vi "MasterAquisitionFile_NoLiveDisplays_IOS.vi"() -> ()   [LabVIEW 2018]
uses:
  <vilib>/userdefined/High Color/IMAQdx.ctl
  <vilib>/vision/driver/IMAQdx.llb/IMAQdx Camera Control Mode.ctl
  <vilib>/vision/driver/IMAQdx.llb/IMAQdx Acquisition Mode.ctl
  <vilib>/vision/driver/IMAQdx.llb/IMAQdx Buffer Number Mode.ctl
  <vilib>/DAQmx/write.llb/DAQmx Write (Digital Bool 1Line 1Point).vi
  <vilib>/DAQmx/read.llb/DAQmx Read (Analog 1D Wfm NChan NSamp).vi
  <vilib>/DAQmx/write.llb/DAQmx Write (Digital 1D Bool NChan 1Samp 1Line).vi
  <vilib>/DAQmx/create/channels.llb/DAQmx Create Channel (DO-Digital Output).vi
  <vilib>/DAQmx/create/channels.llb/DAQmx Create Channel (CO-Pulse Generation-Frequency).vi
  <vilib>/DAQmx/configure/timing.llb/DAQmx Timing (Implicit).vi
  <vilib>/DAQmx/create/channels.llb/DAQmx Create Channel (AI-Voltage-Basic).vi
  <vilib>/DAQmx/configure/timing.llb/DAQmx Timing (Sample Clock).vi
  <vilib>/DAQmx/configure/trigger.llb/DAQmx Start Trigger (Digital Edge).vi
  <vilib>/DAQmx/miscellaneous.llb/DAQmx Fill In Error Info.vi
  <vilib>/vision/driver/NI_Vision_Acquisition_Software.lvlib
  <resource>/objmgr/imaqdx.rc
panel:
  in  "stop":bool
  out "CBV Cam":bool
  out "Pupil Cam":bool
  out "Whisk Cam":bool
  out "Web Cam":bool
  out "Analog Data":bool
  in  "Physical channels":tag="Dev1/ai0:7"
  out "Web Cam Fs":dbl(knob) scale=0.0..200.0
  out "CBV Cam":dbl(knob) scale=0.0..200.0
  out "Whisk Cam Fs":dbl(knob) scale=0.0..200.0
  out "Last Whisk\nBuffer 2":u32=4963
  out "Pupil Cam Fs":dbl(knob) scale=0.0..200.0
  out "Dropped 2":u32(slide) caption="Pupil Cam" scale=0.0..90.0
  in  "Pupil Cam ID":T1="cam2"
  in  "Pupil Cam Trig Source":tag="Dev2/ctr0"
  in  "Exposure Time (microsec)":string="10000"
  out "Solenoids":bool[](array[boolean])
  out "Analog Samples":i32
  in  "Analog Channels":string[](array[string])=["Cortical_LH", "Force_Sensor", "LPadSol", "RPadSol", "AudSol", "Hippocampus", "EMG", "Cortical_RH"]
  in  "Whisker Cam ID":T1="cam1"
  in  "WebCam ID":T1="cam0"
  in  "Analog Acquisition":cluster{"Analog Fs":u16}={"Analog Fs"=20000} {"Analog Fs" format="%0.0f"}
  in  "Camera Acquisition Setup":T2={"CBV Cam Fs"=30, "Whisk Cam Fs"=150, "Web Cam Fs"=15, "Pupil Cam Fs"=30}
  out "Notes Size":i32=7
  out "Notes Reversed":string[](array[string])=["Experimenter", "Animal ID", "Hemisphere", "Solenoid PSI", "Isoflurane time", "Session ID", "Amplifier Gain"]
  out "Notes Array":string[](array[string])=["Amplifier Gain", "Session ID", "Isoflurane time", "Solenoid PSI", "Hemisphere", "Animal ID", "Experimenter"]
  in  "Notes:":T3={"Experimenter"="Kevin", "Animal ID"="T103", "Hemisphere"="Both", "Solenoid PSI"="10", "Isoflurane time"="1000", "Session ID"="Imaging Session One", "Amplifier Gain"="10000"}
  in  "Whisk Cam Trig Source":tag="Dev1/ctr1"
  in  "CBV Cam Trig Source":tag="Dev1/ctr0"
  in  "Left Pad":tag="Dev1/port0/line0"
  in  "Right Pad":tag="Dev1/port0/line1"
  in  "Auditory":tag="Dev1/port0/line2"
  in  "Offset (s)":dbl=15.0
  in  "Duration (s)":dbl=0.1 step=0.1
  in  "Interval (s)":dbl=30.0
  in  "Right Pad":dbl=1.0
  in  "Left Pad":dbl=1.0
  in  "Auditory":dbl=1.0
  in  "Target Path":path=path "D:/T103/Imaging Session One 8.2.19" caption="Final saved file location"
  out "Dropped":u32(slide) caption="Whisk Cam" scale=0.0..450.0
  out "Current file name":string="190412_14_35_08"
  out "CBV Camera":bool
  out "Time Elapsed (Min)":cluster{dbl, dbl}(slide)={15.0, 0.0} scale=0.0..15.0 scale format="%#_2g"
  in  "Time (min)":dbl(knob)=15.0 min=0.5 max=20.0 step=0.5 scale=0.0..20.0 scale format="%#_2g"
  in  "Temp Path":path=path "D:/LabVIEW Streamed Data" caption="Temporary path for streamed data"
  out "Last CBV\nBuffer":i32=9926
  out "Last Whisk\nBuffer":u32=49638
  # "Stimuli"
  # "LPAD"
  # "RPAD"
  # "AUD"
  # "Whisk Cam ID"
  # "Pupil Cam ID"
  # "Ratio"
  # "Web Cam ID"
  # "Data Sampling Rates"
  # "Ratio"
  # "Ratio"
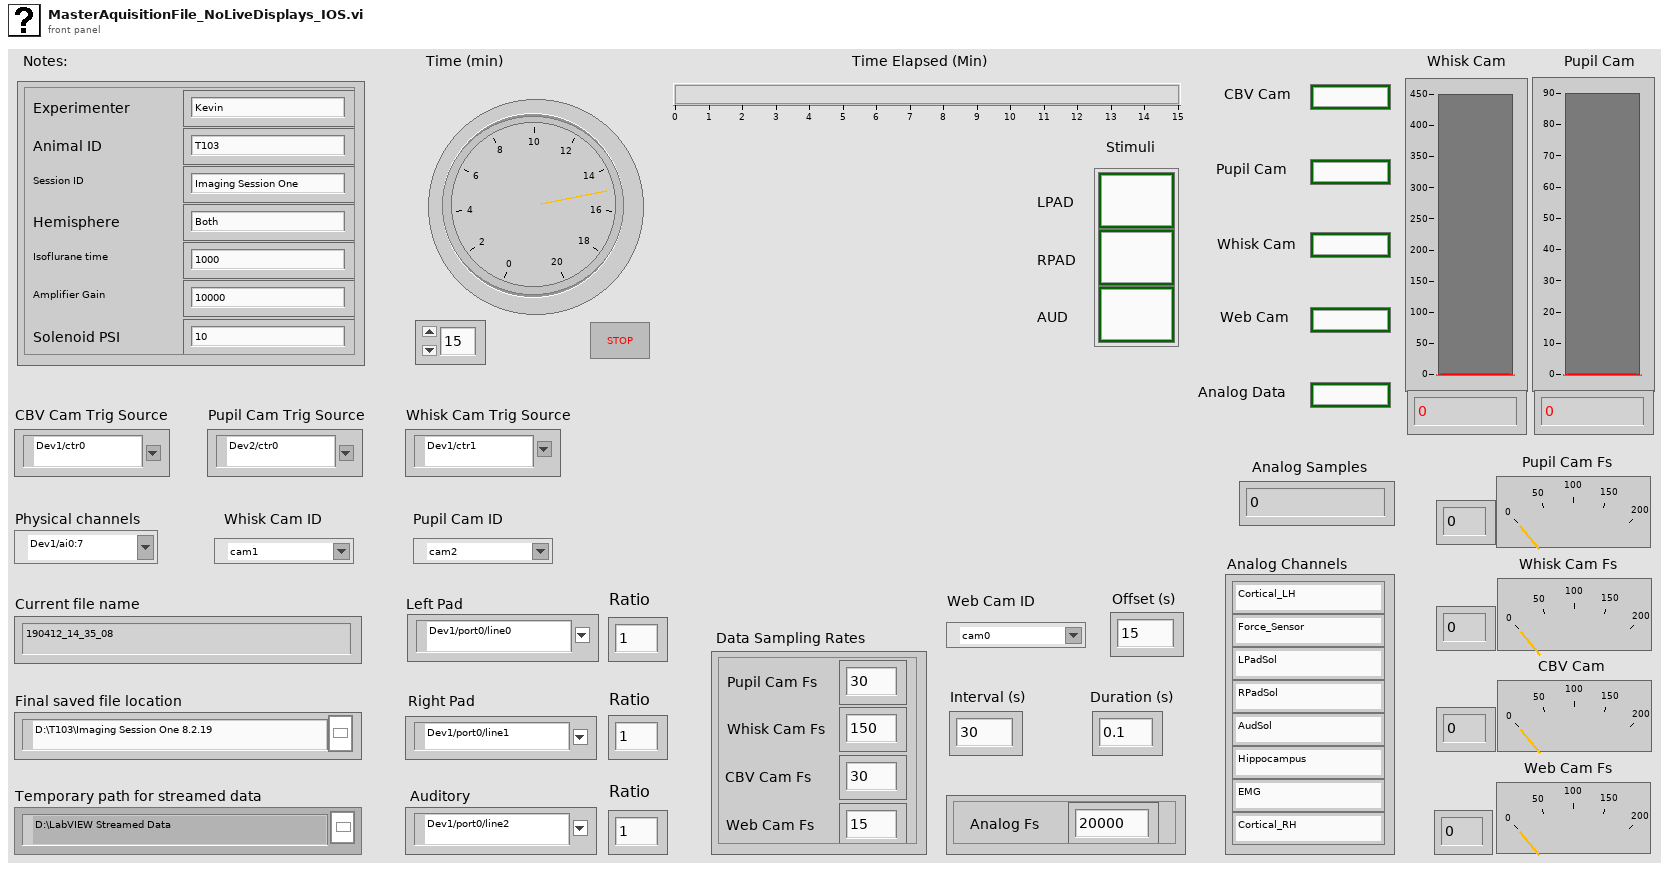
[diagram p1: front panel]
types:
  T1 = typedef "IMAQdx.ctl" = refnum<k21>
  T2 = cluster{"CBV Cam Fs":u16, "Whisk Cam Fs":u16, "Web Cam Fs":u16, "Pupil Cam Fs":u16}
  T3 = cluster{"Experimenter":string, "Animal ID":string, "Hemisphere":string, "Solenoid PSI":string, "Isoflurane time":string, "Session ID":string, "Amplifier Gain":string}
  T4 = enum16{"open", "replace", "create", "open or create", "replace or create", "replace or create with confirmation"}
  T5 = typedef "Image Type" = u32
  T6 = typedef "NI_Vision_Acquisition_Software.lvlib/IMAQdx Acquisition Mode.ctl" = enum32{"One Shot", "Continuous"}
  T7 = typedef "NI_Vision_Acquisition_Software.lvlib/IMAQdx Camera Control Mode.ctl" = enum32{"Controller", "Listener"}
  T8 = enum16{"open", "open or create", "create or replace", "create", "open (read-only)"}
  T9 = typedef "IMAQ AVI2 Refnum.ctl" = refnum<k20>
  T10 = typedef "IMAQ Image.ctl" = refnum<image>
  T11 = enum16{"big-endian, network order", "native, host order", "little-endian"}
  T12 = typedef "NI_Vision_Acquisition_Software.lvlib/IMAQdx Buffer Number Mode.ctl" = enum32{"Next", "Last", "Buffer Number", "Every", "Last New"}
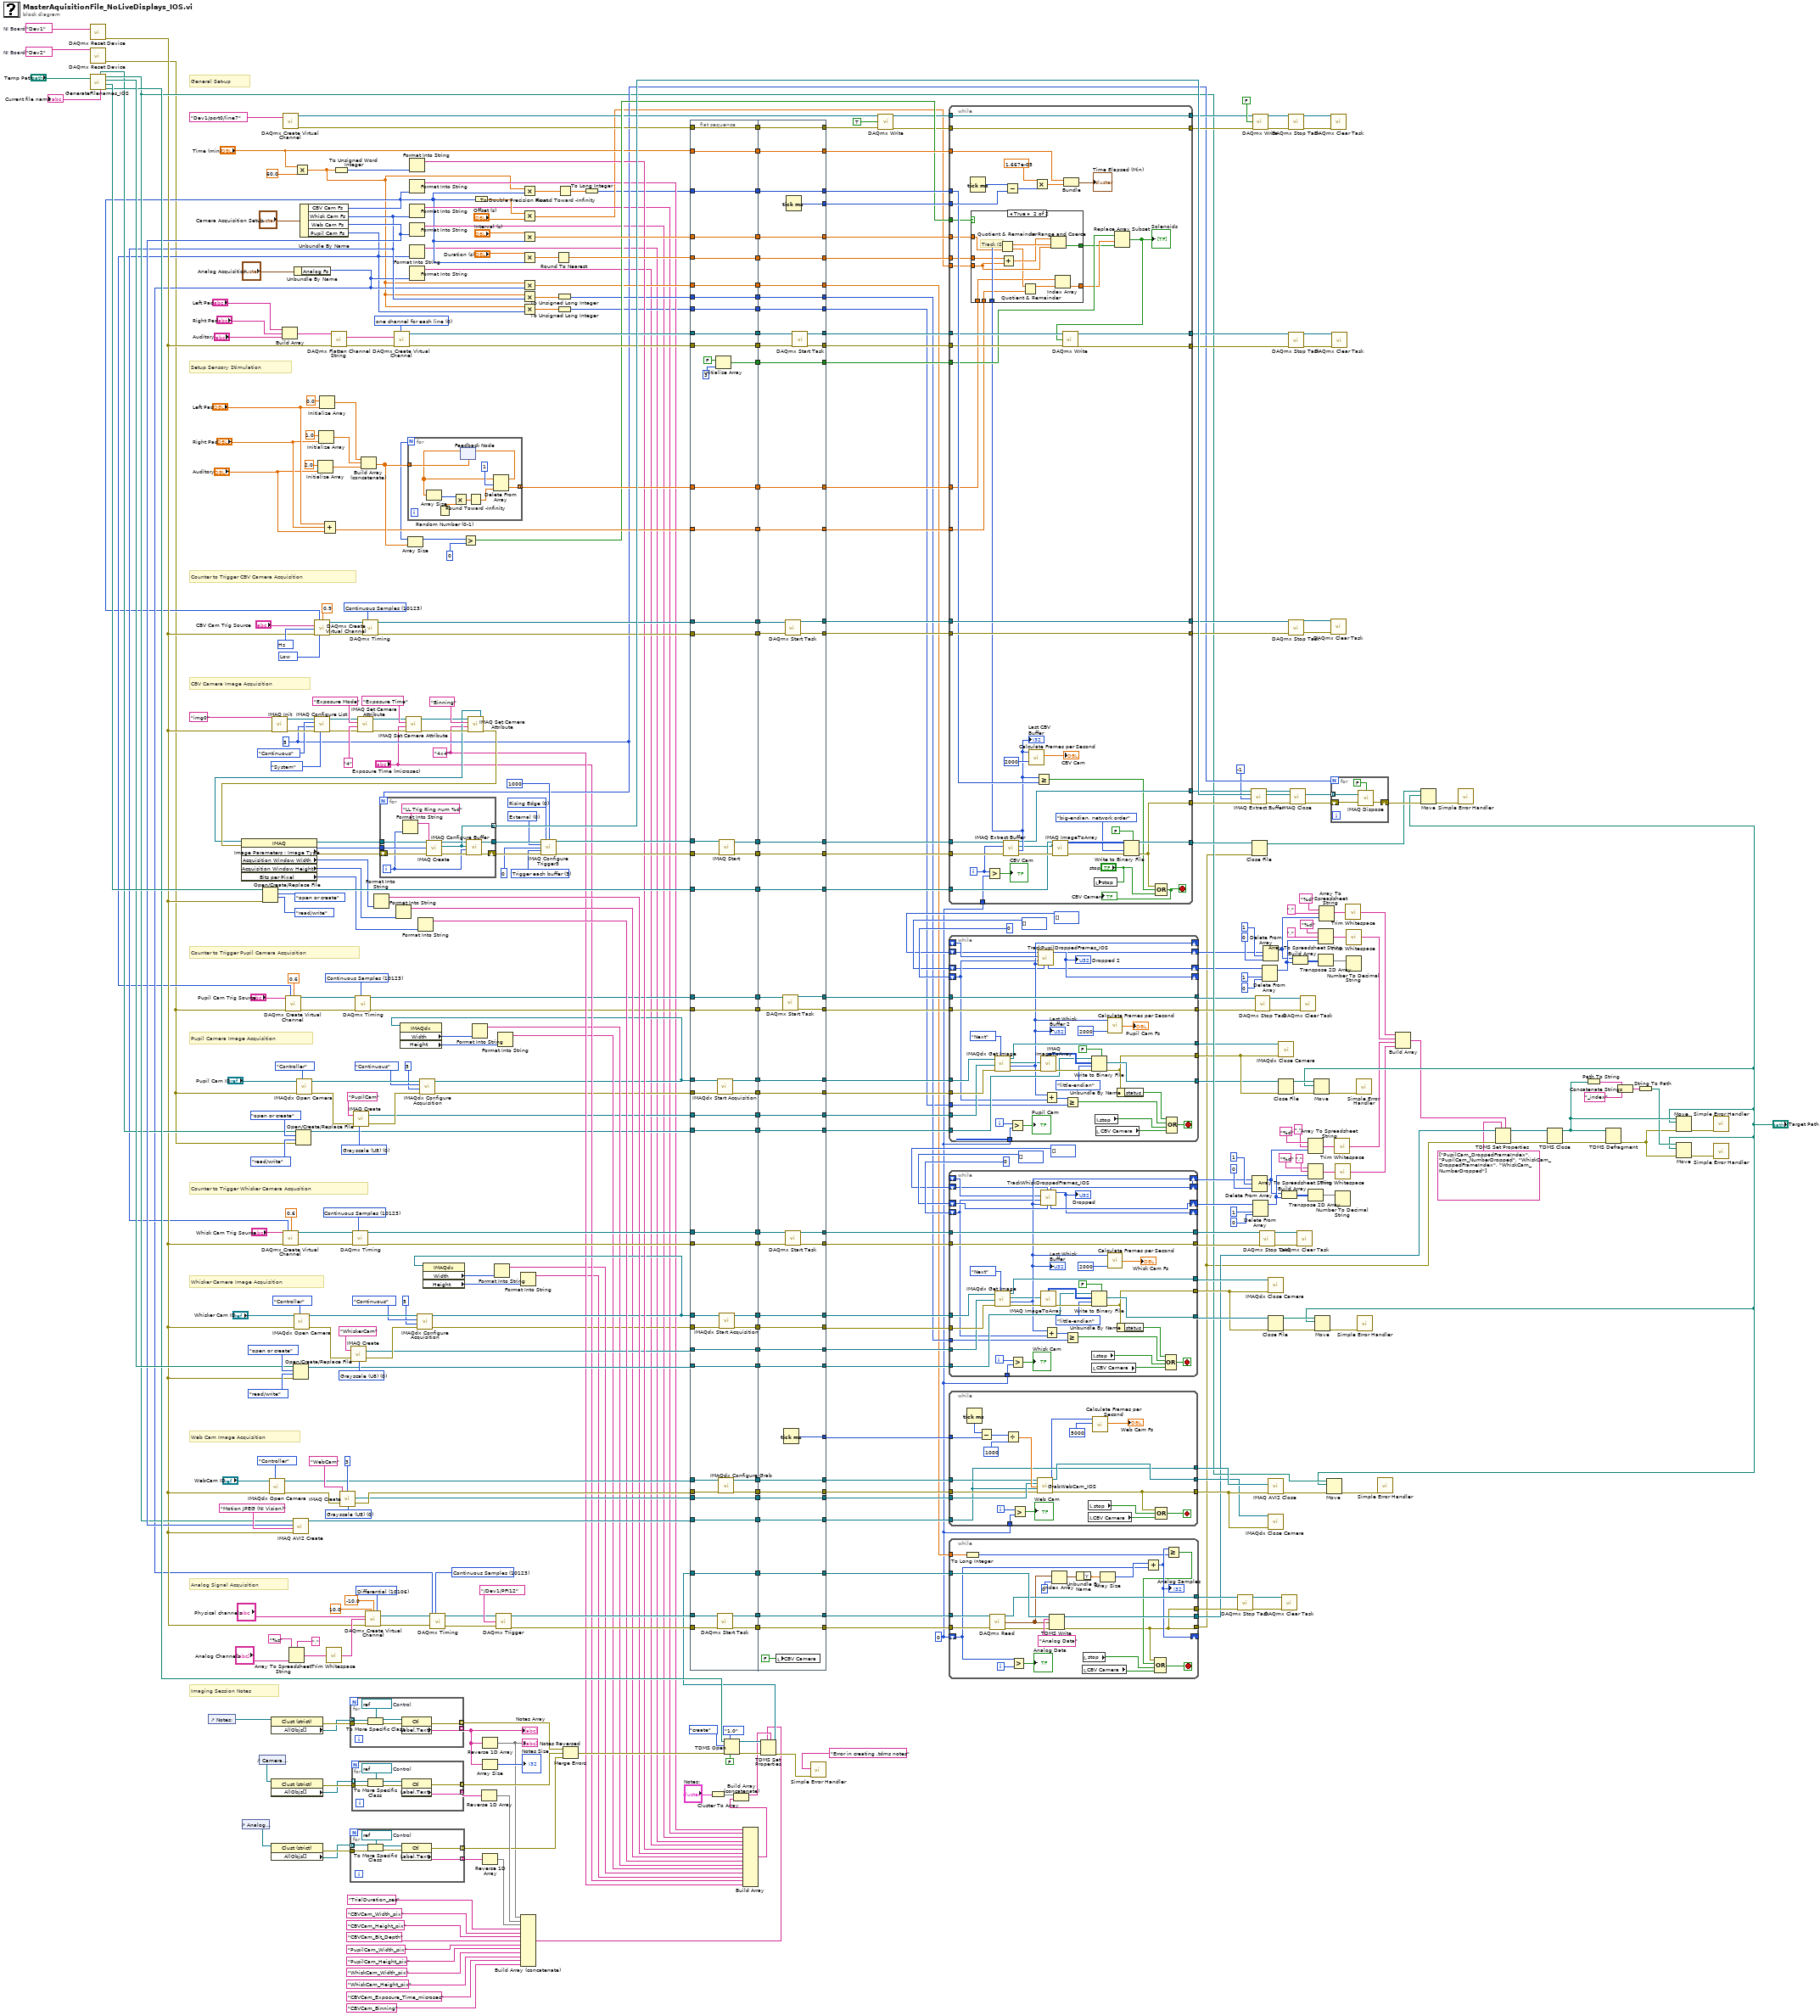
[diagram p0: block diagram]
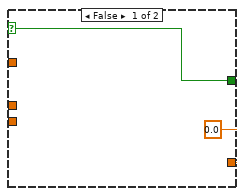
[diagram p2: hidden frame]
diagram:
  w17 = tag "Dev2"  # NI Board
  w108 = 10123 items=["Finite Samples"=10178, "Continuous Samples"=10123, "Hardware Timed Single Point"=12522] ("sample mode")
  w115 = T5 0 items=["Grayscale (U8)", "Grayscale (I16)", "Grayscale (SGL)", "Complex (CSG)", "RGB (U32)", "HSL (U32)", "RGB (U64)", "Grayscale (U16)"] ("Image Type")
  w97 = "4x4" ("Attribute Value")
  w23 = 0
  w281 = 0 items=["one channel for each line", "one channel for all lines"] ("line grouping")
  w334 = 10123 items=["Finite Samples"=10178, "Continuous Samples"=10123, "Hardware Timed Single Point"=12522] ("sample mode")
  w337 = 10106 items=["default"=-1, "RSE"=10083, "NRSE"=10078, "Differential"=10106, "Pseudodifferential"=12529] ("input terminal configuration")
  w388 = T5 0 items=["Grayscale (U8)", "Grayscale (I16)", "Grayscale (SGL)", "Complex (CSG)", "RGB (U32)", "HSL (U32)", "RGB (U64)", "Grayscale (U16)"] ("Image Type")
  w408 = u32 0 items=["Rising Edge", "Falling Edge"] ("Trigger Polarity")
  w411 = u32 0 items=["External"=0, "RTSI"=1, "ISO In"=2, "Scaled Encoder"=5] ("Trigger Type")
  w402 = tag "Dev1"  # NI Board
  w403 = 10123 items=["Finite Samples"=10178, "Continuous Samples"=10123, "Hardware Timed Single Point"=12522] ("sample mode")
  w406 = 10373 items=["Hz"=10373] ("units")
  w407 = 10214 items=["High"=10192, "Low"=10214] ("idle state")
  w127 = u32 5 ("Number of Buffers")
  w409 = u32 3 items=["Disabled", "Trigger start of acquisition", "Trigger start of each buffer list", "Trigger each buffer", "Trigger each line (linescan)", "Trigger end of acquisition"] ("Action")
  w423 = 10123 items=["Finite Samples"=10178, "Continuous Samples"=10123, "Hardware Timed Single Point"=12522] ("sample mode")
  w430 = T5 0 items=["Grayscale (U8)", "Grayscale (I16)", "Grayscale (SGL)", "Complex (CSG)", "RGB (U32)", "HSL (U32)", "RGB (U64)", "Grayscale (U16)"] ("Image Type")
  # "General Set-up"
  # "Pupil Camera Image Acquisition"
  # "Counter to Trigger Pupil Camera Acquisition"
  # "Whisker Camera Image Acquisition"
  # "Imaging Session Notes"
  # "Setup Sensory Stimulation"
  # "CBV Camera Image Acquisition"
  # "Counter to Trigger CBV Camera Acquisition"
  # "Counter to Trigger Whisker Camera Acqusition"
  # "Web Cam Image Acquisition"
  # "Analog Signal Acquisition"
  n1 = call <vilib>:"DAQmx Reset Device.vi"("device in"=w402) -> ("error out"=w82:errorcluster)  [unwired: 14 in]
  n2 = call <vilib>:"DAQmx Reset Device.vi"("device in"=w17) -> ("error out"=w16:errorcluster)  [unwired: 14 in]
  n3 = call "GenerateFilenames_IOS.vi"("path"="Temp Path") -> ("TDMS Path"=w237:path, "Dalsa Path"=w395:path, "Basler Path"=w391:path, "WebCam Path"=w126:path, "Analog file name"=→"Current file name":string, "Basler2 Path"=w106:path)  [unwired: 5 in]
  n4 = control-ref of="Notes:"() -> (w242:refnum<vi>)
  n5 = control-ref of="Analog Acquisition"() -> (w220:refnum<vi>)
  n6 = control-ref of="Camera Acquisition Setup"() -> (w221:refnum<vi>)
  n7 = Open/Create/Replace File(file path (use dialog)=w395, error in=w82, operation (0:open)=T4."open or create", access (0:read/write)=enum16{"read/write", "read-only", "write-only"}."read/write") -> (refnum out=w338:refnum<file>)  [unwired: 2 in, 2 out]
  n8 = call <vilib>:"IMAQdx Open Camera.vi"("Camera Control Mode"=IMAQdx_Camera_Control_Mode."Controller", "error in"=w82, "Session In"="WebCam ID") -> ("error out"=w384:errorcluster, "Session Out"=w382:T1)  [unwired: 7 in]
  n9 = property class="Clust (strict)"(reference=w242) -> (error out=w245:errorcluster, "AllObjs[]"=w134:refnum<vi>[])  [unwired: 1 in, 1 out]
  n10 = property class="Clust (strict)"(reference=w221) -> (error out=w240:errorcluster, "AllObjs[]"=w135:refnum<vi>[])  [unwired: 1 in, 1 out]
  n11 = property class="Clust (strict)"(reference=w220) -> (error out=w219:errorcluster, "AllObjs[]"=w133:refnum<vi>[])  [unwired: 1 in, 1 out]
  n12 = call <vilib>:"IMAQ Init.vi"("error in (no error)"=w82, "Interface Name"="img0") -> ("error out"=w421:errorcluster, "IMAQ Session Out"=w422:refnum<k11>)  [unwired: 8 out]
  n13 = Build Array("Left Pad", "Right Pad", "Auditory") -> (w9:tag[])
  n14 = call-poly <vilib>:"DAQmx Create Virtual Channel.vi"("lines"=tag "Dev1/port0/line7") -> ("task out"=w167:refnum<k21>, "error out"=w170:errorcluster)  [unwired: 13 in]
  n15 = Array To Spreadsheet String(delimiter (Tab)=",", array="Analog Channels", 3:"%s" ("format string")) -> (spreadsheet string=w206:string)
  n16 = Open/Create/Replace File(file path (use dialog)=w391, error in=w82, operation (0:open)=T4."open or create", access (0:read/write)=enum16{"read/write", "read-only", "write-only"}."read/write") -> (refnum out=w356:refnum<file>)  [unwired: 2 in, 2 out]
  n17 = Unbundle By Name("Analog Acquisition") -> ("Analog Fs"=w63:u16)
  n18 = call <vilib>:"IMAQdx Open Camera.vi"("Camera Control Mode"=IMAQdx_Camera_Control_Mode."Controller", "error in"=w82, "Session In"="Whisker Cam ID") -> ("error out"=w433:errorcluster, "Session Out"=w436:T1)  [unwired: 7 in]
  n19 = Multiply(x="Time (min)", y=60.0) -> (x*y=w25:dbl)
  n20 = Open/Create/Replace File(file path (use dialog)=w106, error in=w16, operation (0:open)=T4."open or create", access (0:read/write)=enum16{"read/write", "read-only", "write-only"}."read/write") -> (refnum out=w87:refnum<file>)  [unwired: 2 in, 2 out]
  n21 = call <vilib>:"IMAQdx Open Camera.vi"("Camera Control Mode"=IMAQdx_Camera_Control_Mode."Controller", "error in"=w16, "Session In"="Pupil Cam ID") -> ("error out"=w118:errorcluster, "Session Out"=w121:T1)  [unwired: 7 in]
  n22 = Unbundle By Name("Camera Acquisition Setup") -> ("CBV Cam Fs"=w27:u16, "Whisk Cam Fs"=w68:u16, "Web Cam Fs"=w214:u16, "Pupil Cam Fs"=w61:u16)
  n23 = call-poly <vilib>:"DAQmx Create Virtual Channel.vi"("frequency"=w68, "duty cycle"=0.6, "counter"="Whisk Cam Trig Source", "error in"=w82) -> ("task out"=w425:refnum<k21>, "error out"=w424:errorcluster)  [unwired: 10 in]
  n24 = call-poly <vilib>:"DAQmx Create Virtual Channel.vi"("frequency"=w61, "duty cycle"=0.6, "counter"="Pupil Cam Trig Source", "error in"=w16) -> ("task out"=w110:refnum<k21>, "error out"=w109:errorcluster)  [unwired: 10 in]
  n25 = call "IMAQ AVI2 Create"("error in (no error)"=w82, "Codec"="Motion JPEG (NI Vision)", "Frames Per Second"=w214, "AVI Path"=w126) -> ("AVI Refnum"=w374:T9)  [unwired: 6 in, 1 out]
  n26 = call <vilib>:"IMAQ Configure List.vi"("Memory Location"=enum16{"System", "Onboard"}."System", "error in (no error)"=w421, "Number of buffers"=w127, "Continuous?"=enum16{"One-Shot", "Continuous"}."Continuous" ("Continuous ?"), "IMAQ Session In"=w422) -> ("error out"=w148:errorcluster, "IMAQ Session Out"=w144:refnum<k11>)  [unwired: 1 in, 4 out]
  n27 = call-poly <vilib>:"DAQmx Create Virtual Channel.vi"("frequency"=w27, "duty cycle"=0.9, "counter"="CBV Cam Trig Source", "units"=w406, "error in"=w82, "idle state"=w407) -> ("task out"=w405:refnum<k21>, "error out"=w404:errorcluster)  [unwired: 8 in]
  n28 = Initialize Array(2.0 ("element"), "Auditory") -> (w21:dbl[])
  n29 = Initialize Array(1.0 ("element"), "Right Pad") -> (w285:dbl[])
  n30 = Initialize Array(0.0 ("element"), "Left Pad") -> (w286:dbl[])
  n31 = Compound Arithmetic op=ADD("Left Pad", "Right Pad", "Auditory") -> (w265:dbl)
  n32 = call <vilib>:"Trim Whitespace.vi"("string"=w206) -> ("trimmed string"=w205:string)  [unwired: 1 in]
  n33 = call <vilib>:"DAQmx Flatten Channel String.vi"("names in"=w9, "error in"=w82) -> ("names out"=w247:string, "error out"=w246:errorcluster)  [unwired: 12 in]
  n34 = To Unsigned Word Integer(number=w25) -> (unsigned 16bit integer=w200:u16)
  n35 = call "IMAQ Create"("Border Size"=3, "Image Name"="WebCam", "Image Type"=w388, "error in (no error)"=w384) -> ("New Image"=w381:T10, "error out"=w383:errorcluster)  [unwired: 1 in]
  n36 = for {
    tunnel: [w442] -> w244 mode=indexing
    tunnel: w245 -> [w441]
    tunnel: [w439] -> w228 mode=indexing
    tunnel: w134 -> [w438] mode=indexing
    w443 = refnum<vi> refnum  # Control
    n37 = To More Specific Class(target class=w443, reference=w438, error in=w441) -> (specific class reference=w444:refnum<vi>, error out=w440:errorcluster)
    n38 = property class="Ctl"(reference=w444, error in=w440) -> (error out=w439:errorcluster, "Label.Text"=w442:string)  [unwired: 1 out]
  }
  "Notes Array" <- w244
  n39 = for {
    tunnel: [w449] -> w217 mode=indexing
    tunnel: w219 -> [w448]
    tunnel: [w446] -> w218 mode=indexing
    tunnel: w133 -> [w445] mode=indexing
    w450 = refnum<vi> refnum  # Control
    n40 = To More Specific Class(target class=w450, reference=w445, error in=w448) -> (specific class reference=w451:refnum<vi>, error out=w447:errorcluster)
    n41 = property class="Ctl"(reference=w451, error in=w447) -> (error out=w446:errorcluster, "Label.Text"=w449:string)  [unwired: 1 out]
  }
  n42 = call "IMAQ Create"("Image Name"="WhiskerCam", "Image Type"=w430, "error in (no error)"=w433) -> ("New Image"=w187:T10, "error out"=w431:errorcluster)  [unwired: 2 in]
  n43 = for {
    tunnel: [w456] -> w241 mode=indexing
    tunnel: w240 -> [w455]
    tunnel: [w453] -> w227 mode=indexing
    tunnel: w135 -> [w452] mode=indexing
    w457 = refnum<vi> refnum  # Control
    n44 = To More Specific Class(target class=w457, reference=w452, error in=w455) -> (specific class reference=w458:refnum<vi>, error out=w454:errorcluster)
    n45 = property class="Ctl"(reference=w458, error in=w454) -> (error out=w453:errorcluster, "Label.Text"=w456:string)  [unwired: 1 out]
  }
  n46 = call-poly <vilib>:"DAQmx Timing.vi"("task/channels in"=w425, "sample mode"=w423, "error in"=w424) -> ("task out"=w317:refnum<k21>, "error out"=w315:errorcluster)  [unwired: 11 in]
  n47 = call "IMAQ Create"("Image Name"="PupilCam", "Image Type"=w115, "error in (no error)"=w118) -> ("New Image"=w71:T10, "error out"=w116:errorcluster)  [unwired: 2 in]
  n48 = call-poly <vilib>:"DAQmx Timing.vi"("task/channels in"=w110, "sample mode"=w108, "error in"=w109) -> ("task out"=w85:refnum<k21>, "error out"=w83:errorcluster)  [unwired: 11 in]
  n49 = call <vilib>:"IMAQ Set Camera Attribute.vi"("error in (no error)"=w148, "Attribute Value"="4", "Camera Attribute"="Exposure Mode", "IMAQ Session In"=w144) -> ("error out"=w147:errorcluster, "IMAQ Session Out"=w143:refnum<k11>)  [unwired: 4 in]
  n50 = Build Array (concatenate)(w286, w285, w21) -> (w284:dbl[])
  n51 = call-poly <vilib>:"DAQmx Timing.vi"("task/channels in"=w405, "sample mode"=w403, "error in"=w404) -> ("task out"=w321:refnum<k21>, "error out"=w319:errorcluster)  [unwired: 11 in]
  n52 = call-poly <vilib>:"DAQmx Create Virtual Channel.vi"("maximum value"=10.0, "minimum value"=-10.0, "input terminal configuration"=w337, "physical channels"="Physical channels", "name to assign"=w205, "error in"=w82) -> ("task out"=w336:refnum<k21>, "error out"=w335:errorcluster)  [unwired: 8 in]
  n53 = call-poly <vilib>:"DAQmx Create Virtual Channel.vi"("lines"=w247, "line grouping"=w281, "error in"=w246) -> ("task out"=w279:refnum<k21>, "error out"=w277:errorcluster)  [unwired: 11 in]
  n54 = call <vilib>:"IMAQ Set Camera Attribute.vi"("error in (no error)"=w147, "Attribute Value"="Exposure Time (microsec)", "Camera Attribute"="Exposure Time", "IMAQ Session In"=w143) -> ("error out"=w146:errorcluster, "IMAQ Session Out"=w142:refnum<k11>)  [unwired: 4 in]
  n55 = Array Size(array=w284) -> (size(s)=w211:i32)
  n56 = for {
    N: w211 -> [_]
    tunnel: w284 -> [w462]
    tunnel: [w459] -> w262 mode=concatenating
    n57 = Random Number (0-1)() -> (number: 0 to 1=w466:dbl)
    n58 = feedback #1(w462) -> (w461:dbl[])
    n59 = Array Size(array=w461) -> (size(s)=w467:i32)
    n60 = Multiply(x=w467, y=w466) -> (x*y=w465:dbl)
    n61 = Round Toward -Infinity(1:w465) -> (0:w464:dbl)
    n62 = Delete From Array(array=w461, length=1, index=w464) -> (deleted portion=w459:dbl[], array with subset deleted=w460:dbl[])
    n63 = feedback-in #1(w460) -> ()
  }
  n64 = Format Into String(w200) -> (resulting string=w202:string)  [unwired: 3 in, 1 out]
  n65 = Format Into String(w27) -> (resulting string=w66:string)  [unwired: 3 in, 1 out]
  n66 = Format Into String(w68) -> (resulting string=w65:string)  [unwired: 3 in, 1 out]
  n67 = Format Into String(w214) -> (resulting string=w64:string)  [unwired: 3 in, 1 out]
  n68 = Format Into String(w61) -> (resulting string=w2:string)  [unwired: 3 in, 1 out]
  n69 = Format Into String(w63) -> (resulting string=w1:string)  [unwired: 3 in, 1 out]
  n70 = call <vilib>:"IMAQdx Configure Acquisition.vi"("error in"=w431, "Number of Buffers"=u32 5, "Continuous?"=IMAQdx_Acquisition_Mode."Continuous", "Session In"=w436) -> ("error out"=w24:errorcluster, "Session Out"=w188:T1)  [unwired: 6 in]
  n71 = call <vilib>:"IMAQdx Configure Acquisition.vi"("error in"=w116, "Number of Buffers"=u32 5, "Continuous?"=IMAQdx_Acquisition_Mode."Continuous", "Session In"=w121) -> ("error out"=w89:errorcluster, "Session Out"=w72:T1)  [unwired: 6 in]
  n72 = property class="IMAQdx"(reference=w72) -> ("Width"=w105:u32, "Height"=w104:u32)  [unwired: 1 in, 2 out]
  n73 = property class="IMAQdx"(reference=w188) -> ("Width"=w199:u32, "Height"=w198:u32)  [unwired: 1 in, 2 out]
  n74 = call-poly <vilib>:"DAQmx Timing.vi"("task/channels in"=w336, "sample mode"=w334, "rate"=w63, "error in"=w335) -> ("task out"=w131:refnum<k21>, "error out"=w333:errorcluster)  [unwired: 10 in]
  n75 = Greater?(x=w211, y=0) -> (0:w209:bool)
  n76 = call <vilib>:"IMAQ Set Camera Attribute.vi"("error in (no error)"=w146, "Attribute Value"=w97, "Camera Attribute"="Binning", "IMAQ Session In"=w142) -> ("error out"=w145:errorcluster, "IMAQ Session Out"=w141:refnum<k11>)  [unwired: 4 in]
  n77 = property class="IMAQ"(reference=w141, error in=w145) -> (reference out=w155:refnum<k11>, error out=w154:errorcluster, "Image Parameters : Image Type"=w417:u32, "Acquisition Window Width"=w197:u32, "Acquisition Window Height"=w196:u32, "Bits per Pixel"=w195:u32)
  n78 = Format Into String(w197) -> (resulting string=w194:string)  [unwired: 3 in, 1 out]
  n79 = for {
    N: w127 -> [_]
    tunnel: [w477] -> w413
    tunnel: w417 -> [w475]
    shift-right: [w476] -> w412
    shift-left: w154 -> [w474]
    tunnel: [w469] -> w414 mode=indexing
    tunnel: w155 -> [w468]
    i -> [w470]
    n80 = Format Into String(format string="LL Trig Ring num %d", w470) -> (resulting string=w472:string)  [unwired: 2 in, 1 out]
    n81 = call "IMAQ Create"("Image Name"=w472, "Image Type"=w475, "error in (no error)"=w474) -> ("New Image"=w469:T10, "error out"=w473:errorcluster)  [unwired: 1 in, 1 out]
    n82 = call <vilib>:"IMAQ Configure Buffer.vi"("error in (no error)"=w473, "Buffer Number"=w470, "Image In"=w469, "IMAQ Session In"=w468) -> ("error out"=w476:errorcluster, "IMAQ Session Out"=w477:refnum<k11>)  [unwired: 2 in, 4 out]
  }
  n83 = Format Into String(w196) -> (resulting string=w128:string)  [unwired: 3 in, 1 out]
  n84 = Format Into String(w195) -> (resulting string=w193:string)  [unwired: 3 in, 1 out]
  n85 = Format Into String(w105) -> (resulting string=w92:string)  [unwired: 3 in, 1 out]
  n86 = To Double Precision Float(number=w27) -> (double precision float=w248:dbl)
  n87 = Reverse 1D Array(array=w241) -> (reversed array=w231:string[])
  n88 = Reverse 1D Array(array=w244) -> (reversed array=w132:string[])
  "Notes Reversed" <- w132
  n89 = Array Size(array=w244) -> (size(s)=→"Notes Size":i32)
  n90 = Reverse 1D Array(array=w217) -> (reversed array=w216:string[])
  n91 = Format Into String(w199) -> (resulting string=w94:string)  [unwired: 3 in, 1 out]
  n92 = call-poly <vilib>:"DAQmx Trigger.vi"("task/channels in"=w131, "source"=tag "/Dev1/PFI12", "error in"=w333) -> ("task out"=w331:refnum<k21>, "error out"=w330:errorcluster)  [unwired: 11 in]
  n93 = Format Into String(w104) -> (resulting string=w93:string)  [unwired: 3 in, 1 out]
  n94 = Build Array (concatenate)(w132, w231, w216, "TrialDuration_sec", "CBVCam_Width_pix", "CBVCam_Height_pix", "CBVCam_Bit_Depth", "PupilCam_Width_pix", "PupilCam_Height_pix", "WhiskCam_Width_pix", "WhiskCam_Height_pix", "CBVCam_Exposure_Time_microsec" ("element"), "CBVCam_Binning" ("element")) -> (w123:string[])
  n95 = Format Into String(w198) -> (resulting string=w95:string)  [unwired: 3 in, 1 out]
  n96 = Multiply(x=w25, y=w27) -> (x*y=w393:dbl)
  n97 = Multiply(x="Offset (s)", y=w248) -> (x*y=w59:dbl)
  n98 = Multiply(x="Interval (s)", y=w27) -> (x*y=w269:dbl)
  n99 = Multiply(x="Duration (s)", y=w27) -> (x*y=w256:dbl)
  n100 = Multiply(x=w25, y=w63) -> (x*y=w176:dbl)
  n101 = Multiply(x=w68, y=w25) -> (x*y=w129:dbl)
  n102 = Multiply(x=w61, y=w25) -> (x*y=w67:dbl)
  n103 = call <vilib>:"IMAQ Configure Trigger3.vi"("IMAQ Session In"=w413, "Polarity"=w408, "Frame timeout (ms)"=u32 1000 ("Frame Timeout (ms)"), "Type"=w411, "Line Number"=u32 0 ("Trigger Line Number"), "Action"=w409, "error in (no error)"=w412) -> ("IMAQ Session Out"=w355:refnum<k11>, "error out"=w354:errorcluster)  [unwired: 2 in, 5 out]
  n104 = Round To Nearest(number=w256) -> (nearest integer value=w255:dbl)
  n105 = To Unsigned Long Integer(number=w129) -> (unsigned 32bit integer=w174:u32)
  n106 = To Unsigned Long Integer(number=w67) -> (unsigned 32bit integer=w62:u32)
  n107 = Round Toward -Infinity(1:w393) -> (0:w392:dbl)
  n108 = Merge Errors(w228, w227, w218) -> (w226:errorcluster)
  n109 = To Long Integer(number=w392) -> (32bit integer=w26:i32)
  n110 = flat-sequence {
    tunnel: w383 -> [w526]
    tunnel: w382 -> [w525]
    tunnel: w381 -> [w524]
    tunnel: [w524] -> w380
    tunnel: [w523] -> w378
    tunnel: [w522] -> w376
    tunnel: w374 -> [w521]
    tunnel: [w521] -> w373
    tunnel: w188 -> [w520]
    tunnel: w24 -> [w519]
    tunnel: [w518] -> w363
    tunnel: [w517] -> w361
    tunnel: [w516] -> w359
    tunnel: w187 -> [w516]
    tunnel: [w515] -> w357
    tunnel: w356 -> [w515]
    tunnel: w355 -> [w514]
    tunnel: w354 -> [w513]
    tunnel: [w512] -> w352
    tunnel: [w511] -> w350
    tunnel: w26 -> [w510]
    tunnel: [w510] -> w344
    tunnel: "Time (min)" -> [w509]
    tunnel: [w509] -> w341
    tunnel: [w508] -> w339
    tunnel: w338 -> [w508]
    tunnel: w331 -> [w507]
    tunnel: w330 -> [w506]
    tunnel: [w505] -> w329
    tunnel: [w504] -> w328
    tunnel: [w503] -> w323
    tunnel: w229 -> [w503]
    tunnel: w321 -> [w502]
    tunnel: [w502] -> w320
    tunnel: w319 -> [w501]
    tunnel: [w501] -> w318
    tunnel: w317 -> [w500]
    tunnel: [w500] -> w316
    tunnel: w315 -> [w499]
    tunnel: [w499] -> w314
    tunnel: w279 -> [w498]
    tunnel: [w498] -> w280
    tunnel: w277 -> [w497]
    tunnel: [w497] -> w278
    tunnel: w269 -> [w496]
    tunnel: [w496] -> w268
    tunnel: [w495] -> w266
    tunnel: w255 -> [w495]
    tunnel: w265 -> [w494]
    tunnel: [w494] -> w264
    tunnel: w262 -> [w493]
    tunnel: [w493] -> w261
    tunnel: [w491] -> w259
    tunnel: w176 -> [w489]
    tunnel: [w489] -> w175
    tunnel: w174 -> [w488]
    tunnel: [w488] -> w173
    tunnel: w170 -> [w487]
    tunnel: [w487] -> w169
    tunnel: [w480] -> w91
    tunnel: w72 -> [w481]
    tunnel: [w478] -> w90
    tunnel: w89 -> [w479]
    tunnel: [w486] -> w88
    tunnel: w87 -> [w486]
    tunnel: [w485] -> w86
    tunnel: w85 -> [w485]
    tunnel: [w484] -> w84
    tunnel: w83 -> [w484]
    tunnel: w71 -> [w483]
    tunnel: [w483] -> w70
    tunnel: w62 -> [w482]
    tunnel: [w482] -> w60
    tunnel: [w574] -> w385
    tunnel: w380 -> [w573]
    tunnel: [w573] -> w379
    tunnel: w378 -> [w572]
    tunnel: [w572] -> w377
    tunnel: w376 -> [w571]
    tunnel: [w571] -> w375
    tunnel: w373 -> [w570]
    tunnel: [w570] -> w372
    tunnel: [w552] -> w369
    tunnel: [w551] -> w367
    tunnel: [w569] -> w364
    tunnel: w363 -> [w569]
    tunnel: [w568] -> w362
    tunnel: w361 -> [w568]
    tunnel: [w567] -> w360
    tunnel: w359 -> [w567]
    tunnel: [w566] -> w358
    tunnel: w357 -> [w566]
    tunnel: [w565] -> w353
    tunnel: w352 -> [w565]
    tunnel: [w564] -> w351
    tunnel: w350 -> [w564]
    tunnel: [w556] -> w348
    tunnel: [w555] -> w346
    tunnel: [w563] -> w345
    tunnel: w344 -> [w562]
    tunnel: [w562] -> w343
    tunnel: [w561] -> w342
    tunnel: w341 -> [w561]
    tunnel: [w560] -> w340
    tunnel: w339 -> [w560]
    tunnel: [w559] -> w326
    tunnel: w329 -> [w559]
    tunnel: [w558] -> w327
    tunnel: w328 -> [w558]
    tunnel: [w557] -> w324
    tunnel: w323 -> [w557]
    tunnel: w320 -> [w554]
    tunnel: w318 -> [w553]
    tunnel: w316 -> [w550]
    tunnel: w314 -> [w549]
    tunnel: w280 -> [w548]
    tunnel: w278 -> [w547]
    tunnel: [w546] -> w276
    tunnel: [w545] -> w275
    tunnel: [w544] -> w270
    tunnel: w268 -> [w544]
    tunnel: [w543] -> w267
    tunnel: w266 -> [w543]
    tunnel: w264 -> [w542]
    tunnel: [w542] -> w263
    tunnel: w261 -> [w541]
    tunnel: [w541] -> w260
    tunnel: w259 -> [w540]
    tunnel: [w540] -> w258
    tunnel: w175 -> [w539]
    tunnel: [w539] -> w56
    tunnel: w173 -> [w538]
    tunnel: [w538] -> w58
    tunnel: w169 -> [w537]
    tunnel: [w537] -> w168
    tunnel: w91 -> [w535]
    tunnel: w90 -> [w534]
    tunnel: w88 -> [w533]
    tunnel: w86 -> [w530]
    tunnel: w84 -> [w529]
    tunnel: [w527] -> w78
    tunnel: [w528] -> w77
    tunnel: [w535] -> w76
    tunnel: [w534] -> w75
    tunnel: [w533] -> w74
    tunnel: [w532] -> w69
    tunnel: w70 -> [w532]
    tunnel: [w531] -> w57
    tunnel: w60 -> [w531]
    frame #0 {
      n111 = Initialize Array(FALSE, 3 ("dimension size")) -> (w491:bool[])
      n112 = call <vilib>:"IMAQdx Start Acquisition.vi"("error in"=w479, "Session In"=w481) -> ("error out"=w478:errorcluster, "Session Out"=w480:T1)  [unwired: 8 in]
      n113 = call <vilib>:"DAQmx Start Task.vi"("task/channels in"=w507, "error in"=w506) -> ("task out"=w505:refnum<k21>, "error out"=w504:errorcluster)  [unwired: 12 in]
      n114 = call <vilib>:"IMAQdx Configure Grab.vi"("error in"=w526, "Session In"=w525) -> ("error out"=w522:errorcluster, "Session Out"=w523:T1)  [unwired: 8 in]
      n115 = call <vilib>:"IMAQ Start.vi"("error in (no error)"=w513, "IMAQ Session In"=w514) -> ("error out"=w511:errorcluster, "IMAQ Session Out"=w512:refnum<k11>)  [unwired: 8 out]
      n116 = call <vilib>:"IMAQdx Start Acquisition.vi"("error in"=w519, "Session In"=w520) -> ("error out"=w517:errorcluster, "Session Out"=w518:T1)  [unwired: 8 in]
    }
    frame #1 {
      n117 = local write "CBV Camera"(FALSE ("Finished Acquiring")) -> ()
      n118 = call <vilib>:"DAQmx Start Task.vi"("task/channels in"=w530, "error in"=w529) -> ("task out"=w527:refnum<k21>, "error out"=w528:errorcluster)  [unwired: 12 in]
      n119 = Tick Count (ms)() -> (millisecond timer value=w574:u32)
      n120 = call <vilib>:"DAQmx Start Task.vi"("task/channels in"=w554, "error in"=w553) -> ("task out"=w556:refnum<k21>, "error out"=w555:errorcluster)  [unwired: 12 in]
      n121 = call <vilib>:"DAQmx Start Task.vi"("task/channels in"=w550, "error in"=w549) -> ("task out"=w552:refnum<k21>, "error out"=w551:errorcluster)  [unwired: 12 in]
      n122 = Tick Count (ms)() -> (millisecond timer value=w563:u32)
      n123 = call <vilib>:"DAQmx Start Task.vi"("task/channels in"=w548, "error in"=w547) -> ("task out"=w546:refnum<k21>, "error out"=w545:errorcluster)  [unwired: 12 in]
    }
  }
  n124 = Cluster To Array(cluster="Notes:") -> (array=w238:string[])
  n125 = TDMS Open(6:FALSE ("disable buffering? (T)"), 7:enum16{"1.0", "2.0"}."1.0" ("file format version (2.0)"), 8:w226, 10:T8."create" ("operation (0:open)"), 11:w237) -> (0:w232:errorcluster, 3:w233:refnum<k34>)  [unwired: 2 in]
  n126 = Build Array(w66, w65, w64, w2, w1, w202, w194, w128, w193, w92, w93, w94, w95, "Exposure Time (microsec)", w97) -> (w213:string[])
  n127 = Build Array (concatenate)(w238, w213) -> (w230:string[])
  n128 = TDMS Set Properties(5:w230, 7:w123, 8:w232, 11:w233) -> (0:w225:errorcluster, 3:w229:refnum<k34>)  [unwired: 2 in, 2 out]
  n129 = call <vilib>:"Simple Error Handler.vi"("error source (\" \")"="Error in creating .tdms notes" ("error source (\" \")"), "error in (no error)"=w225) -> ()  [unwired: 3 in, 5 out]
  n130 = call-poly <vilib>:"DAQmx Write.vi"("task/channels in"=w167, "data"=TRUE, "error in"=w168) -> ("task out"=w165:refnum<k21>, "error out"=w163:errorcluster)  [unwired: 10 in, 1 out]
  n131 = while {
    tunnel: w353 -> [w620]
    tunnel: w351 -> [w621]
    tunnel: [w585] -> w397
    tunnel: [w583] -> w398
    tunnel: [w615] -> w396
    tunnel: [w610] -> w349
    tunnel: w348 -> [w610]
    tunnel: [w609] -> w347
    tunnel: w346 -> [w609]
    tunnel: w345 -> [w608]
    tunnel: w343 -> [w607]
    tunnel: w342 -> [w606]
    tunnel: w340 -> [w582]
    tunnel: w276 -> [w603]
    tunnel: w275 -> [w602]
    tunnel: [w601] -> w274
    tunnel: [w600] -> w273
    tunnel: w270 -> [w595]
    tunnel: w267 -> [w594]
    tunnel: w263 -> [w592]
    tunnel: w260 -> [w590]
    tunnel: w258 -> [w599]
    tunnel: w59 -> [w593]
    tunnel: w209 -> [w597]
    tunnel: w165 -> [w587]
    tunnel: [w587] -> w164
    tunnel: [w586] -> w162
    tunnel: w163 -> [w586]
    tunnel: w23 -> [w577]
    i -> [w578]
    stop <- w588 stop-if-true
    # "Track ISI"
    n132 = Tick Count (ms)() -> (millisecond timer value=w613:u32)
    n133 = Greater?(x=w578, y=w577) -> (0:→"CBV Cam":bool)
    n134 = call <vilib>:"IMAQ Extract Buffer.vi"("error in (no error)"=w621, "Buffer to extract"=w578, "IMAQ Session In"=w620) -> ("error out"=w614:errorcluster, "Buffer Number"=w596:i32, "Image Out"=w575:T10, "IMAQ Session Out"=w583:refnum<k11>)  [unwired: 5 out]
    "Last CBV\nBuffer" <- w596
    n135 = case shown="True" w597 {
      selector: w597 -> [w623 _]
      tunnel: w596 -> [_ w633]
      tunnel: w595 -> [_ w632]
      tunnel: w594 -> [_ w631]
      tunnel: w593 -> [_ w630]
      tunnel: w592 -> [_ w627]
      tunnel: [0.0 ("element") w624] -> w591
      tunnel: w590 -> [_ w626]
      tunnel: [w623 w625] -> w589
      frame False {
      }
      frame True {
        n136 = Quotient & Remainder(x=w633, y=w632) -> (x-y*floor(x/y)=w635:dbl, floor(x/y)=w628:dbl)
        n137 = Add(x=w631, y=w630) -> (x+y=w634:dbl)
        n138 = Quotient & Remainder(x=w628, y=w627) -> (x-y*floor(x/y)=w629:dbl)  [unwired: 1 out]
        n139 = In Range and Coerce(upper limit=w634, x=w635, lower limit=w630) -> (In Range?=w625:bool)  [unwired: 1 out]
        n140 = Index Array(array=w626, index=w629) -> (element=w624:dbl)
      }
    }
    n141 = Subtract(x=w613, y=w608) -> (x-y=w612:u32)
    n142 = call <vilib>:"Calculate Frames per Second.vi"("Update Interval (ms)"=u32 2000, "Buffer Number"=w596) -> ("Processed Frames/s"=→"CBV Cam":dbl)  [unwired: 7 in, 2 out]
    n143 = Multiply(x=w612, y=1.667e-05) -> (x*y=w611:dbl)
    n144 = Greater Or Equal?(x=w596, y=w607) -> (x >= y?=w581:bool)
    n145 = call "IMAQ ImageToArray"("error in (no error)"=w614, "Image"=w575) -> ("error out"=w619:errorcluster, "Image Pixels (I16)"=w618:i16[][])  [unwired: 2 in, 3 out]
    n146 = Bundle("Time (min)"=w606, w611) -> (→"Time Elapsed (Min)":cluster{"Time (min)":dbl, dbl})  [unwired: 1 in]
    n147 = local write "stop"("stop") -> ()
    n148 = Replace Array Subset(array=w599, new element=w589, index=w591) -> (w598:bool[])
    "Solenoids" <- w598
    n149 = call-poly <vilib>:"DAQmx Write.vi"("task/channels in"=w603, "data"=w598, "error in"=w602) -> ("task out"=w601:refnum<k21>, "error out"=w600:errorcluster)  [unwired: 10 in, 1 out]
    n150 = Write to Binary File(file (use dialog)=w582, data=w618, error in=w619, 5:FALSE ("prepend array or string size? (T)"), 9:T11."big-endian, network order" ("byte order (0:big-endian, network order)")) -> (refnum out=w615:refnum<file>, error out=w585:errorcluster)  [unwired: 1 in, 1 out]
    n151 = Compound Arithmetic op=OR(w585, w581, "stop") -> (w588:bool)
    "CBV Camera" <- w588
  }
  n152 = while {
    tunnel: w78 -> [w662]
    tunnel: [w663] -> w41
    tunnel: w77 -> [w663]
    tunnel: [w662] -> w40
    tunnel: [w651] -> w38
    tunnel: [w652] -> w39
    tunnel: [w661] -> w37
    tunnel: w76 -> [w660]
    tunnel: w75 -> [w659]
    tunnel: w69 -> [w658]
    tunnel: w74 -> [w657]
    shift-right: [w650] -> _
    shift-left: _ -> [w656]
    shift-right: [w655] -> _
    shift-left: u32 0 ("New Lost") -> [w649]
    shift-right: [w654] -> w35
    shift-left: u32[] [] ("NewBuffNum") -> [w643]
    shift-right: [w653] -> w36
    shift-left: u32[] [] ("NewNumLost") -> [w644]
    tunnel: w57 -> [w642]
    tunnel: w23 -> [w639]
    i -> [w640]
    stop <- w645 stop-if-true
    n153 = call <vilib>:"IMAQdx Get Image.vi"("Buffer Number Mode (Next)"=IMAQdx_Buffer_Number_Mode."Next", "error in"=w659, "Image In"=w658, "Session In"=w660) -> ("error out"=w670:errorcluster, "Buffer Number Out"=w650:u32, "Image Out"=w636:T10, "Session Out"=w651:T1)  [unwired: 4 in]
    "Last Whisk\nBuffer 2" <- w650
    n154 = Greater?(x=w640, y=w639) -> (0:→"Pupil Cam":bool)
    n155 = call "TrackPupilDroppedFrames_IOS.vi"("NumLost"=w644, "BuffNum"=w643, "Curr Buffer"=w650, "Prev Lost"=w649, "Prev Buffer"=w656) -> ("New Lost"=w655:u32, "NewNumLost"=w653:u32[], "NewBuffNum"=w654:u32[])  [unwired: 4 in]
    "Dropped 2" <- w655
    n156 = call "IMAQ ImageToArray"("error in (no error)"=w670, "Image"=w636) -> ("error out"=w669:errorcluster, "Image Pixels (U8)"=w668:u8[][])  [unwired: 2 in, 3 out]
    n157 = Add(x=w650, y=w649) -> (x+y=w648:u32)
    n158 = Greater Or Equal?(x=w648, y=w642) -> (x >= y?=w646:bool)
    n159 = Write to Binary File(file (use dialog)=w657, data=w668, error in=w669, 5:FALSE ("prepend array or string size? (T)"), 9:T11."little-endian" ("byte order (0:big-endian, network order)")) -> (refnum out=w661:refnum<file>, error out=w652:errorcluster)  [unwired: 1 in, 1 out]
    n160 = local read "stop"() -> (w638:bool)
    n161 = local read "CBV Camera"() -> (w637:bool)
    n162 = call <vilib>:"Calculate Frames per Second.vi"("Update Interval (ms)"=u32 2000, "Buffer Number"=w650) -> ("Processed Frames/s"=→"Pupil Cam Fs":dbl)  [unwired: 7 in, 2 out]
    n163 = Unbundle By Name(w652) -> ("status"=w647:bool)
    n164 = Compound Arithmetic op=OR(w647, w646, w638, w637) -> (w645:bool)
  }
  n165 = while {
    tunnel: w369 -> [w699]
    tunnel: [w700] -> w368
    tunnel: w367 -> [w700]
    tunnel: [w699] -> w366
    tunnel: [w692] -> w185
    tunnel: [w693] -> w249
    tunnel: [w698] -> w365
    tunnel: w364 -> [w697]
    tunnel: w362 -> [w696]
    tunnel: w360 -> [w695]
    tunnel: w358 -> [w694]
    shift-right: [w680] -> _
    shift-left: _ -> [w678]
    shift-right: [w675] -> _
    shift-left: u32 0 ("New Lost") -> [w679]
    shift-right: [w676] -> w177
    shift-left: u32[] [] ("NewBuffNum") -> [w677]
    shift-right: [w682] -> w308
    shift-left: u32[] [] ("NewNumLost") -> [w681]
    tunnel: w58 -> [w690]
    tunnel: w23 -> [w683]
    i -> [w684]
    stop <- w687 stop-if-true
    n166 = call <vilib>:"IMAQdx Get Image.vi"("Buffer Number Mode (Next)"=IMAQdx_Buffer_Number_Mode."Next", "error in"=w696, "Image In"=w695, "Session In"=w697) -> ("error out"=w706:errorcluster, "Buffer Number Out"=w680:u32, "Image Out"=w672:T10, "Session Out"=w692:T1)  [unwired: 4 in]
    "Last Whisk\nBuffer" <- w680
    n167 = Greater?(x=w684, y=w683) -> (0:→"Whisk Cam":bool)
    n168 = call "IMAQ ImageToArray"("error in (no error)"=w706, "Image"=w672) -> ("error out"=w705:errorcluster, "Image Pixels (U8)"=w704:u8[][])  [unwired: 2 in, 3 out]
    n169 = call "TrackWhiskDroppedFrames_IOS.vi"("NumLost"=w681, "BuffNum"=w677, "Curr Buffer"=w680, "Prev Lost"=w679, "Prev Buffer"=w678) -> ("New Lost"=w675:u32, "NewNumLost"=w682:u32[], "NewBuffNum"=w676:u32[])  [unwired: 4 in]
    "Dropped" <- w675
    n170 = Add(x=w680, y=w679) -> (x+y=w691:u32)
    n171 = Greater Or Equal?(x=w691, y=w690) -> (x >= y?=w688:bool)
    n172 = Write to Binary File(file (use dialog)=w694, data=w704, error in=w705, 5:FALSE ("prepend array or string size? (T)"), 9:T11."little-endian" ("byte order (0:big-endian, network order)")) -> (refnum out=w698:refnum<file>, error out=w693:errorcluster)  [unwired: 1 in, 1 out]
    n173 = local read "stop"() -> (w674:bool)
    n174 = local read "CBV Camera"() -> (w673:bool)
    n175 = call <vilib>:"Calculate Frames per Second.vi"("Update Interval (ms)"=u32 2000, "Buffer Number"=w680) -> ("Processed Frames/s"=→"Whisk Cam Fs":dbl)  [unwired: 7 in, 2 out]
    n176 = Unbundle By Name(w693) -> ("status"=w689:bool)
    n177 = Compound Arithmetic op=OR(w689, w688, w674, w673) -> (w687:bool)
  }
  n178 = while {
    tunnel: w385 -> [w723]
    tunnel: w379 -> [w721]
    tunnel: w377 -> [w720]
    tunnel: w375 -> [w719]
    tunnel: w372 -> [w717]
    tunnel: [w718] -> w73
    tunnel: [w709] -> w370
    tunnel: [w717] -> w371
    tunnel: w23 -> [w712]
    i -> [w713]
    stop <- w710 stop-if-true
    n179 = Tick Count (ms)() -> (millisecond timer value=w725:u32)
    n180 = Subtract(x=w725, y=w723) -> (x-y=w726:u32)
    n181 = Divide(x=w726, y=u32 1000) -> (x/y=w722:dbl)
    n182 = Greater?(x=w713, y=w712) -> (0:→"Web Cam":bool)
    n183 = call "GrabWebCam_IOS.vi"("Session In"=w720, "Image In"=w721, "Trial Time"=w722, "AVI Refnum"=w717, "error in"=w719) -> ("Session Out"=w718:T1, "Buffer Number Out"=w716:u32, "error out"=w709:errorcluster)  [unwired: 7 in, 1 out]
    n184 = local read "CBV Camera"() -> (w711:bool)
    n185 = local read "stop"() -> (w708:bool)
    n186 = call <vilib>:"Calculate Frames per Second.vi"("Update Interval (ms)"=u32 5000, "Buffer Number"=w716) -> ("Processed Frames/s"=→"Web Cam Fs":dbl)  [unwired: 7 in, 2 out]
    n187 = Compound Arithmetic op=OR(w709, w708, w711) -> (w710:bool)
  }
  n188 = while {
    tunnel: w327 -> [w750]
    tunnel: w326 -> [w749]
    tunnel: w324 -> [w748]
    tunnel: [w747] -> w29
    tunnel: [w735] -> w28
    tunnel: [w746] -> w322
    shift-right: [w739] -> _
    shift-left: w23 -> [w730]
    tunnel: [w735] -> w124
    tunnel: w56 -> [w733]
    i -> [w731]
    stop <- w736 stop-if-true
    n189 = To Long Integer(number=w733) -> (32bit integer=w734:i32)
    n190 = call-poly <vilib>:"DAQmx Read.vi"("task/channels in"=w749, "error in"=w750) -> ("task out"=w746:refnum<k21>, "data"=w744:waveform(dbl)[], "error out"=w738:errorcluster)  [unwired: 11 in]
    n191 = Greater?(x=w730, y=w731) -> (0:→"Analog Data":bool)
    n192 = TDMS Write(0:w748, 5:"Analog Data" ("group name in (Untitled)"), 9:w744, 11:w738) -> (4:w747:refnum<k34>, 15:w735:errorcluster)  [unwired: 2 in, 2 out]
    n193 = Index Array(array=w744, index=0) -> (element=w742:waveform(dbl))
    n194 = Unbundle By Name(w742) -> ("Y"=w741:dbl[])
    n195 = local read "CBV Camera"() -> (w729:bool)
    n196 = local read "stop"() -> (w728:bool)
    n197 = Array Size(array=w741) -> (size(s)=w740:i32)
    n198 = Add(x=w740, y=w730) -> (x+y=w739:i32)
    "Analog Samples" <- w739
    n199 = Greater Or Equal?(x=w739, y=w734) -> (x >= y?=w737:bool)
    n200 = Compound Arithmetic op=OR(w735, w737, w728, w729) -> (w736:bool)
  }
  n201 = call <vilib>:"DAQmx Stop Task.vi"("task/channels in"=w322, "error in"=w124) -> ("task out"=w251:refnum<k21>, "error out"=w250:errorcluster)  [unwired: 12 in]
  n202 = call <vilib>:"IMAQ Extract Buffer.vi"("error in (no error)"=w397, "Buffer to extract"=-1, "IMAQ Session In"=w398) -> ("error out"=w419:errorcluster, "IMAQ Session Out"=w418:refnum<k11>)  [unwired: 7 out]
  n203 = Close File(refnum=w396, error in=w28) -> (path=w302:path)  [unwired: 1 out]
  n204 = Delete From Array(array=w177, length=1, index=0) -> (array with subset deleted=w137:u32[])  [unwired: 1 out]
  n205 = call-poly <vilib>:"DAQmx Write.vi"("task/channels in"=w164, "data"=FALSE, "error in"=w162) -> ("task out"=w161:refnum<k21>, "error out"=w159:errorcluster)  [unwired: 10 in, 1 out]
  n206 = Delete From Array(array=w308, length=1, index=0) -> (array with subset deleted=w138:u32[])  [unwired: 1 out]
  n207 = call <vilib>:"DAQmx Stop Task.vi"("task/channels in"=w40, "error in"=w41) -> ("task out"=w12:refnum<k21>, "error out"=w13:errorcluster)  [unwired: 12 in]
  n208 = call <vilib>:"DAQmx Stop Task.vi"("task/channels in"=w366, "error in"=w368) -> ("task out"=w10:refnum<k21>, "error out"=w11:errorcluster)  [unwired: 12 in]
  n209 = Delete From Array(array=w36, length=1, index=0) -> (array with subset deleted=w43:u32[])  [unwired: 1 out]
  n210 = Delete From Array(array=w35, length=1, index=0) -> (array with subset deleted=w42:u32[])  [unwired: 1 out]
  n211 = call <vilib>:"IMAQdx Close Camera.vi"("error in"=w249, "Session In"=w185) -> ()  [unwired: 9 in, 1 out]
  n212 = Close File(refnum=w365, error in=w249) -> (path=w300:path, error out=w299:errorcluster)
  n213 = call "IMAQ AVI2 Close"("error in (no error)"=w370, "AVI Refnum"=w371) -> ("error out"=w301:errorcluster)  [unwired: 9 in]
  n214 = call <vilib>:"IMAQdx Close Camera.vi"("error in"=w370, "Session In"=w73) -> ()  [unwired: 9 in, 1 out]
  n215 = call <vilib>:"IMAQdx Close Camera.vi"("error in"=w39, "Session In"=w38) -> ()  [unwired: 9 in, 1 out]
  n216 = Close File(refnum=w37, error in=w39) -> (path=w32:path, error out=w31:errorcluster)
  n217 = Build Array(w137, w138) -> (w140:u32[][])
  n218 = call <vilib>:"DAQmx Clear Task.vi"("task in"=w251, "error in"=w250) -> ()  [unwired: 13 in, 1 out]
  n219 = call <vilib>:"DAQmx Stop Task.vi"("task/channels in"=w161, "error in"=w159) -> ("task out"=w160:refnum<k21>, "error out"=w158:errorcluster)  [unwired: 12 in]
  n220 = call <vilib>:"DAQmx Stop Task.vi"("task/channels in"=w274, "error in"=w273) -> ("task out"=w272:refnum<k21>, "error out"=w271:errorcluster)  [unwired: 12 in]
  n221 = call <vilib>:"DAQmx Stop Task.vi"("task/channels in"=w349, "error in"=w347) -> ("task out"=w14:refnum<k21>, "error out"=w15:errorcluster)  [unwired: 12 in]
  n222 = call <vilib>:"IMAQ Close.vi"("error in (no error)"=w419, "IMAQ Session In"=w418) -> ("error out"=w420:errorcluster)  [unwired: 9 out]
  n223 = Build Array(w42, w43) -> (w45:u32[][])
  n224 = call <vilib>:"DAQmx Clear Task.vi"("task in"=w10, "error in"=w11) -> ()  [unwired: 13 in, 1 out]
  n225 = call <vilib>:"DAQmx Clear Task.vi"("task in"=w12, "error in"=w13) -> ()  [unwired: 13 in, 1 out]
  n226 = Array To Spreadsheet String(delimiter (Tab)=",", array=w138, 3:"%d" ("format string")) -> (spreadsheet string=w178:string)
  n227 = Transpose 2D Array(2D array=w140) -> (transposed array=w139:u32[][])
  n228 = Array To Spreadsheet String(delimiter (Tab)=",", array=w137, 3:"%d" ("format string")) -> (spreadsheet string=w179:string)
  n229 = Move(source path=w32, error in=w31, 10:"Target Path") -> (error out=w33:errorcluster)  [unwired: 2 in, 2 out]
  n230 = Move(source path=w300, error in=w299, 10:"Target Path") -> (error out=w297:errorcluster)  [unwired: 2 in, 2 out]
  n231 = Array To Spreadsheet String(delimiter (Tab)=",", array=w43, 3:"%d" ("format string")) -> (spreadsheet string=w46:string)
  n232 = Transpose 2D Array(2D array=w45) -> (transposed array=w44:u32[][])
  n233 = Array To Spreadsheet String(delimiter (Tab)=",", array=w42, 3:"%d" ("format string")) -> (spreadsheet string=w47:string)
  n234 = Move(source path=w126, error in=w301, 10:"Target Path") -> (error out=w296:errorcluster)  [unwired: 2 in, 2 out]
  n235 = call <vilib>:"DAQmx Clear Task.vi"("task in"=w14, "error in"=w15) -> ()  [unwired: 13 in, 1 out]
  n236 = call <vilib>:"DAQmx Clear Task.vi"("task in"=w160, "error in"=w158) -> ()  [unwired: 13 in, 1 out]
  n237 = for {
    N: w127 -> [_]
    tunnel: w414 -> [w754] mode=indexing
    shift-right: [w752] -> w304
    shift-left: w420 -> [w753]
    n238 = call "IMAQ Dispose"("All Images? (No)"=FALSE, "Image"=w754, "error in (no error)"=w753) -> ("error out"=w752:errorcluster)  [unwired: 3 out]
  }
  n239 = call <vilib>:"DAQmx Clear Task.vi"("task in"=w272, "error in"=w271) -> ()  [unwired: 13 in, 1 out]
  n240 = call <vilib>:"Trim Whitespace.vi"("string"=w179) -> ("trimmed string"=w5:string)  [unwired: 1 in]
  n241 = call <vilib>:"Trim Whitespace.vi"("string"=w178) -> ("trimmed string"=w4:string)  [unwired: 1 in]
  n242 = Number To Decimal String(number=w139) -> ()  [unwired: 1 in, 1 out]
  n243 = call <vilib>:"Trim Whitespace.vi"("string"=w47) -> ("trimmed string"=w6:string)  [unwired: 1 in]
  n244 = call <vilib>:"Trim Whitespace.vi"("string"=w46) -> ("trimmed string"=w7:string)  [unwired: 1 in]
  n245 = Number To Decimal String(number=w44) -> ()  [unwired: 1 in, 1 out]
  n246 = call <vilib>:"Simple Error Handler.vi"("error in (no error)"=w33) -> ()  [unwired: 1 in, 8 out]
  n247 = call <vilib>:"Simple Error Handler.vi"("error in (no error)"=w297) -> ()  [unwired: 1 in, 8 out]
  n248 = call <vilib>:"Simple Error Handler.vi"("error in (no error)"=w296) -> ()  [unwired: 1 in, 8 out]
  n249 = Build Array(w6, w7, w5, w4) -> (w3:string[])
  n250 = Move(source path=w302, error in=w304, 10:"Target Path") -> (error out=w303:errorcluster)  [unwired: 2 in, 2 out]
  n251 = call <vilib>:"Simple Error Handler.vi"("error in (no error)"=w303) -> ()  [unwired: 1 in, 8 out]
  n252 = TDMS Set Properties(5:w3, 7:string[] ["PupilCam_DroppedFrameIndex", "PupilCam_NumberDropped", "WhiskCam_DroppedFrameIndex", "WhiskCam_NumberDropped"] ("channel name(s) in (Untitled)"), 8:w28, 11:w29) -> (0:w186:errorcluster, 3:w184:refnum<k34>)  [unwired: 2 in, 2 out]
  n253 = TDMS Close(8:w186, 11:w184) -> (0:w305:errorcluster, 3:w293:path)
  n254 = Path To String(path=w293) -> (string=w295:string)
  n255 = TDMS Defragment(4:w305, 7:w293) -> (0:w290:errorcluster)
  n256 = Concatenate Strings(w295, "_index" ("string")) -> (w292:string)
  n257 = String To Path(string=w292) -> (path=w291:path)
  n258 = Move(source path=w293, error in=w290, 10:"Target Path") -> (error out=w298:errorcluster)  [unwired: 2 in, 2 out]
  n259 = Move(source path=w291, error in=w290, 10:"Target Path") -> (error out=w34:errorcluster)  [unwired: 2 in, 2 out]
  n260 = call <vilib>:"Simple Error Handler.vi"("error in (no error)"=w298) -> ()  [unwired: 1 in, 8 out]
  n261 = call <vilib>:"Simple Error Handler.vi"("error in (no error)"=w34) -> ()  [unwired: 1 in, 8 out]
